vi "SerialCom_main.vi"(0 "VISA resource name":refnum<visa-resource-name>, 5 "write buffer":string, 11 "error in (no error)":errorcluster) -> (15 "error out":errorcluster)   [LabVIEW 2018]
uses:
  <vilib>/Instr/_visa.llb/VISA Flush IO Buffer Mask.ctl
  <vilib>/Instr/_visa.llb/VISA Configure Serial Port (Instr).vi
panel:
  out "binary[7]":string
  out "number[7]":u32
  out "byte[7]":string
  out "number[4]":u32
  out "number[5]":u32
  out "number[6]":u32
  out "binary[6]":string
  out "byte[6]":string
  out "binary[5]":string
  out "byte[5]":string
  out "byte[4]":string
  out "binary[4]":string
  in  "resetValues":bool
  out "binary[3]":string
  out "number[3]":u32
  out "byte[3]":string
  out "number[0]":u32
  out "number[1]":u32
  out "number[2]":u32
  out "binary[2]":string
  out "byte[2]":string
  out "binary[1]":string
  out "byte[1]":string
  out "byte[0]":string
  out "binary[0]":string
  out "byte Array":string[](array[string])
  out "valid byte":string
  out "bytes at port":u32
  out "byte count":u32
  out "read buffer":string
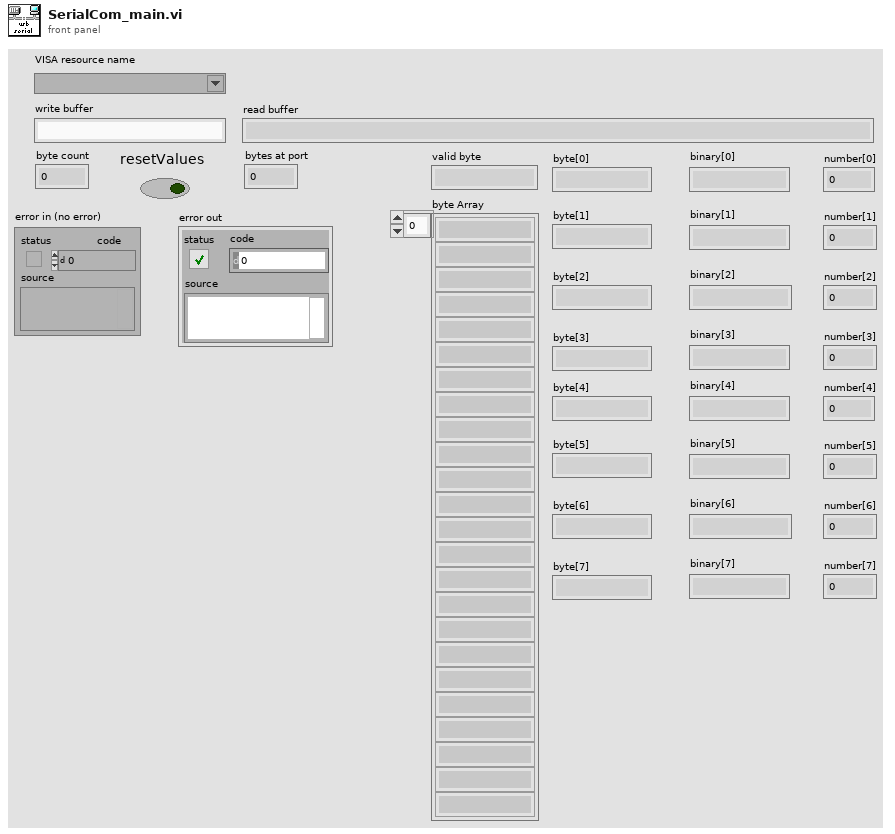
[diagram p1: front panel]
types:
  T1 = typedef "VISA Flush IO Buffer Mask.ctl" = u16
  T2 = cluster{"[0]":string, "[1]":string, "[2]":string, "[3]":string, "[4]":string, "[5]":string, "[6]":string, "[7]":string, "[8]":string}
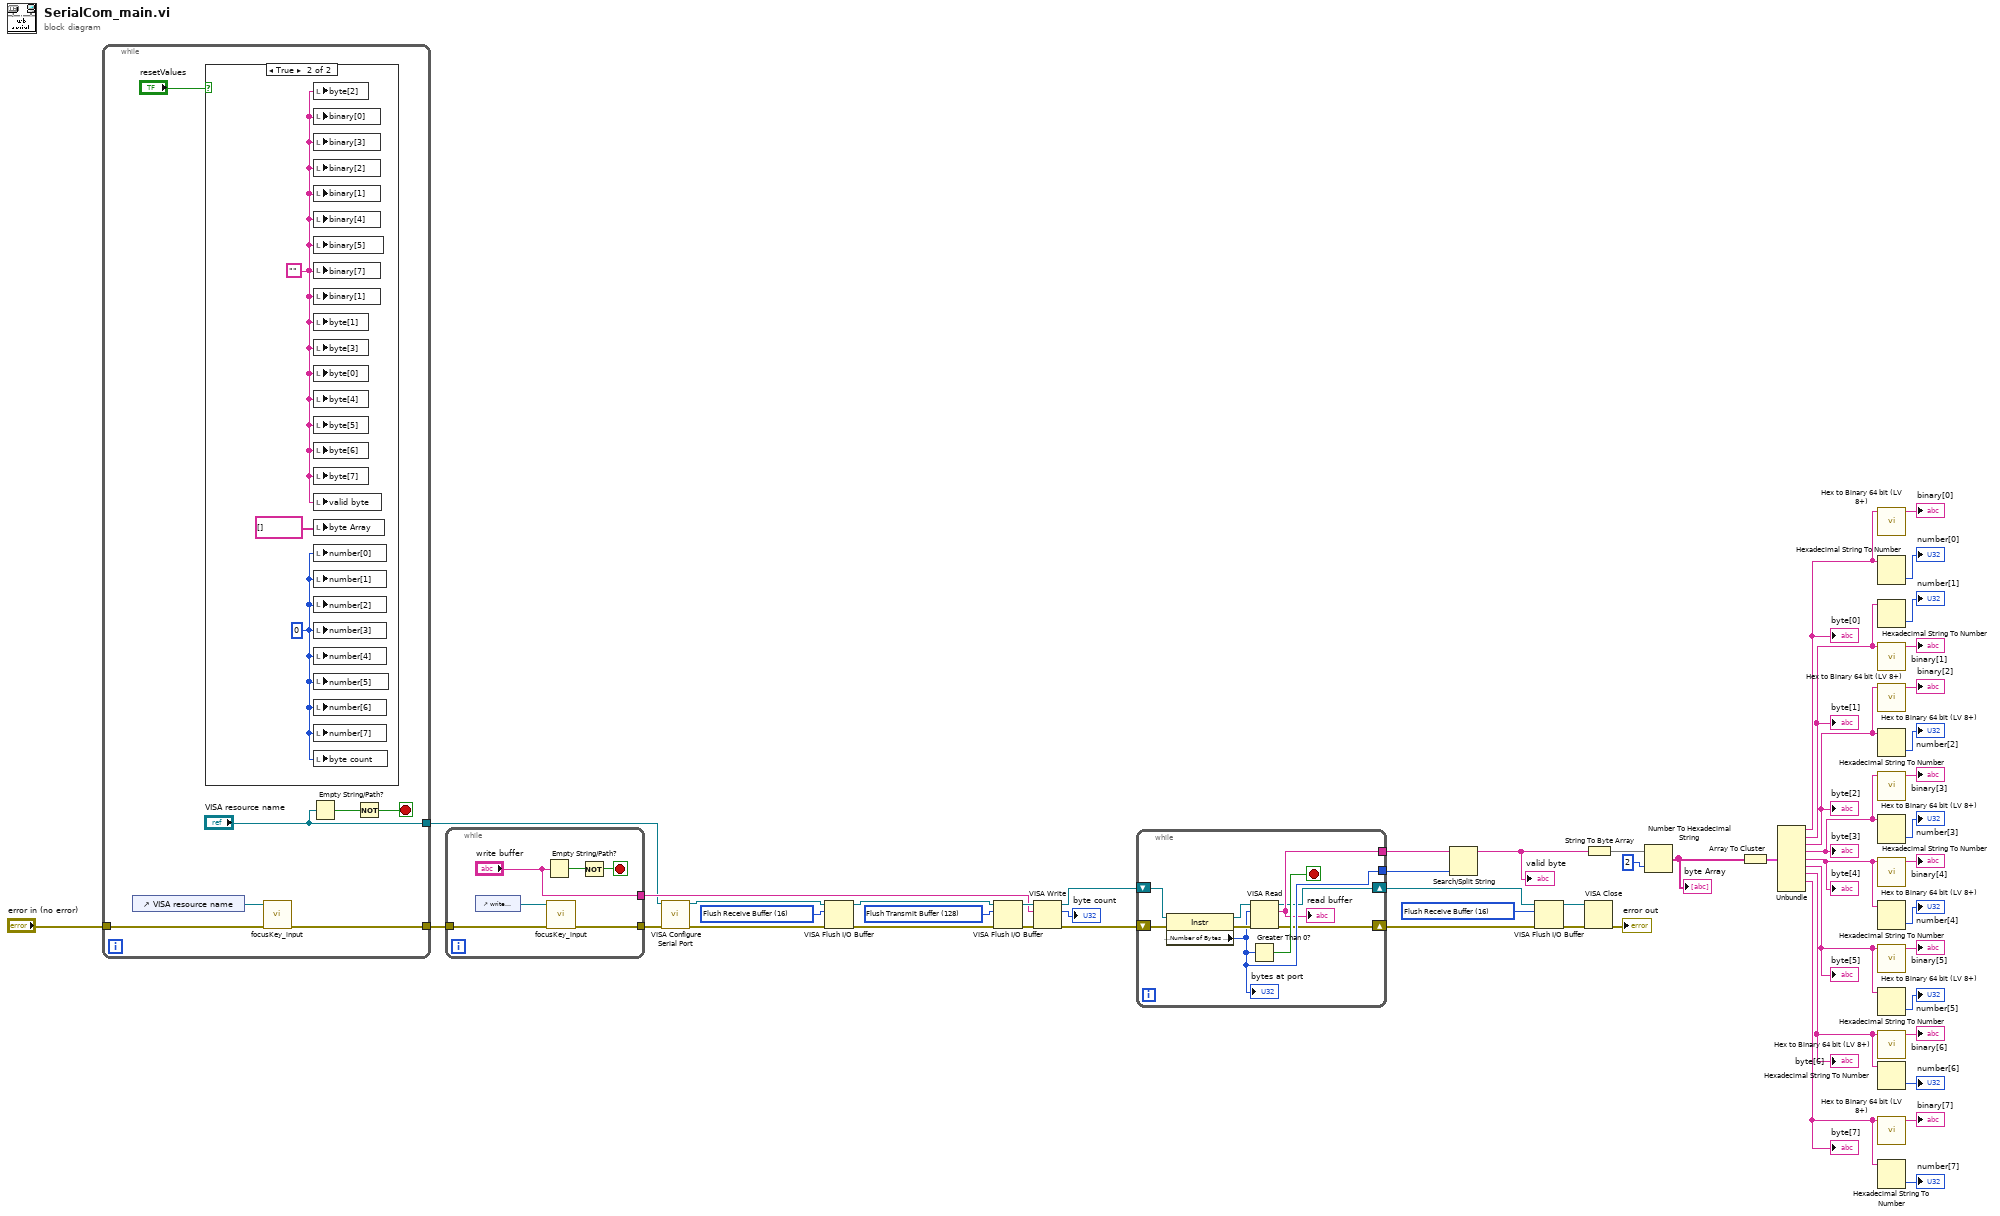
[diagram p0: block diagram]
diagram:
  w36 = T1 128 items=["Flush Receive Buffer"=16, "Write Transmit Buffer to Device"=32, "Flush Receive Buffer (No I/O)"=64, "Flush Transmit Buffer"=128] ("Mask")
  w40 = T1 16 items=["Flush Receive Buffer"=16, "Write Transmit Buffer to Device"=32, "Flush Receive Buffer (No I/O)"=64, "Flush Transmit Buffer"=128] ("Mask")
  w43 = T1 16 items=["Flush Receive Buffer"=16, "Write Transmit Buffer to Device"=32, "Flush Receive Buffer (No I/O)"=64, "Flush Transmit Buffer"=128] ("Mask")
  n1 = while {
    tunnel: ["VISA resource name"] -> w29
    tunnel: [w60] -> w28
    tunnel: "error in (no error)" -> [w59]
    stop <- w55 stop-if-true
    n2 = control-ref of="VISA resource name"() -> (w58:refnum<vi>)
    n3 = case shown="True" "resetValues" {
      frame False {
      }
      frame True {
        w62 = u32 0
        w61 = ""
        n4 = local write "byte[2]"(w61) -> ()
        n5 = local write "binary[0]"(w61) -> ()
        n6 = local write "binary[3]"(w61) -> ()
        n7 = local write "binary[2]"(w61) -> ()
        n8 = local write "binary[1]"(w61) -> ()
        n9 = local write "binary[4]"(w61) -> ()
        n10 = local write "binary[5]"(w61) -> ()
        n11 = local write "binary[7]"(w61) -> ()
        n12 = local write "binary[1]"(w61) -> ()
        n13 = local write "byte[1]"(w61) -> ()
        n14 = local write "byte[3]"(w61) -> ()
        n15 = local write "byte[0]"(w61) -> ()
        n16 = local write "byte[4]"(w61) -> ()
        n17 = local write "byte[5]"(w61) -> ()
        n18 = local write "byte[6]"(w61) -> ()
        n19 = local write "byte[7]"(w61) -> ()
        n20 = local write "valid byte"(w61) -> ()
        n21 = local write "byte Array"(string[] []) -> ()
        n22 = local write "number[0]"(w62) -> ()
        n23 = local write "number[1]"(w62) -> ()
        n24 = local write "number[2]"(w62) -> ()
        n25 = local write "number[3]"(w62) -> ()
        n26 = local write "number[4]"(w62) -> ()
        n27 = local write "number[5]"(w62) -> ()
        n28 = local write "number[6]"(w62) -> ()
        n29 = local write "number[7]"(w62) -> ()
        n30 = local write "byte count"(w62) -> ()
      }
    }
    n31 = call "focusKey_input.vi"("error in (no error)"=w59, "reference"=w58) -> ("error out"=w60:errorcluster)  [unwired: 9 in]
    n32 = Empty String/Path?(string/path="VISA resource name") -> (empty?=w56:bool)
    n33 = Not(x=w56) -> (.not. x?=w55:bool)
  }
  n34 = while {
    tunnel: ["write buffer"] -> w30
    tunnel: w28 -> [w69]
    tunnel: [w68] -> w27
    stop <- w64 stop-if-true
    n35 = control-ref of="write buffer"() -> (w67:refnum<vi>)
    n36 = Empty String/Path?(string/path="write buffer") -> (empty?=w65:bool)
    n37 = call "focusKey_input.vi"("error in (no error)"=w69, "reference"=w67) -> ("error out"=w68:errorcluster)  [unwired: 9 in]
    n38 = Not(x=w65) -> (.not. x?=w64:bool)
  }
  n39 = call-poly "VISA Configure Serial Port"("VISA resource name"=w29, "error in (no error)"=w27) -> ("VISA resource name out"=w42:refnum<visa-resource-name>, "error out"=w41:errorcluster)  [unwired: 12 in]
  n40 = VISA Flush I/O Buffer(VISA resource name=w42, mask (16)=w40, error in (no error)=w41) -> (VISA resource name out=w37:refnum<visa-resource-name>, error out=w38:errorcluster)
  n41 = VISA Flush I/O Buffer(VISA resource name=w37, mask (16)=w36, error in (no error)=w38) -> (VISA resource name out=w35:refnum<visa-resource-name>, error out=w34:errorcluster)
  n42 = VISA Write(VISA resource name=w35, write buffer=w30, error in (no error)=w34) -> (VISA resource name out=w53:refnum<visa-resource-name>, return count=→"byte count":u32, error out=w52:errorcluster)
  n43 = while {
    tunnel: [w72] -> w50
    tunnel: [w73] -> w47
    shift-right: [w70] -> w39
    shift-left: w53 -> [w78]
    shift-right: [w71] -> w44
    shift-left: w52 -> [w77]
    stop <- w74 stop-if-true
    n44 = property class="Instr"(reference=w78, error in=w77) -> (reference out=w75:refnum<visa-resource-name>, error out=w76:errorcluster, "Serial Settings:Number of Bytes at Serial Port"=w73:u32)
    "bytes at port" <- w73
    n45 = Greater Than 0?(x=w73) -> (x > 0?=w74:bool)
    n46 = VISA Read(VISA resource name=w75, byte count=w73, error in (no error)=w76) -> (VISA resource name out=w70:refnum<visa-resource-name>, read buffer=w72:string, error out=w71:errorcluster)  [unwired: 1 out]
    "read buffer" <- w72
  }
  n47 = Search/Split String(string=w50, offset (0)=w47) -> (substring before match=w45:string)  [unwired: 1 in, 2 out]
  "valid byte" <- w45
  n48 = VISA Flush I/O Buffer(VISA resource name=w39, mask (16)=w43, error in (no error)=w44) -> (VISA resource name out=w33:refnum<visa-resource-name>, error out=w32:errorcluster)
  n49 = String To Byte Array(string=w45) -> (unsigned byte array=w49:u8[])
  n50 = VISA Close(VISA resource name=w33, error in (no error)=w32) -> (error out=→"error out":errorcluster)
  n51 = Number To Hexadecimal String(1:i16 2 ("width (-)"), 2:w49) -> (0:w48:string[])
  "byte Array" <- w48
  n52 = Array To Cluster(array=w48) -> (cluster=w15:T2)
  n53 = Unbundle(w15) -> ("[0]"=w16:string, "[1]"=w17:string, "[2]"=w23:string, "[3]"=w13:string, "[4]"=w8:string, "[5]"=w7:string, "[6]"=w6:string, "[7]"=w5:string)  [unwired: 1 out]
  "byte[0]" <- w16
  "byte[1]" <- w17
  "byte[2]" <- w23
  "byte[3]" <- w13
  "byte[4]" <- w8
  "byte[5]" <- w7
  "byte[6]" <- w6
  "byte[7]" <- w5
  n54 = call "Hex to Binary 64 bit (LV 8+).vi"("Hexadecimal String"=w16) -> ("Binary String"=→"binary[0]":string)  [unwired: 6 in, 2 out]
  n55 = Hexadecimal String To Number(string=w16) -> (number=→"number[0]":u32)  [unwired: 2 in, 1 out]
  n56 = Hexadecimal String To Number(string=w17) -> (number=→"number[1]":u32)  [unwired: 2 in, 1 out]
  n57 = call "Hex to Binary 64 bit (LV 8+).vi"("Hexadecimal String"=w17) -> ("Binary String"=→"binary[1]":string)  [unwired: 6 in, 2 out]
  n58 = call "Hex to Binary 64 bit (LV 8+).vi"("Hexadecimal String"=w23) -> ("Binary String"=→"binary[2]":string)  [unwired: 6 in, 2 out]
  n59 = Hexadecimal String To Number(string=w23) -> (number=→"number[2]":u32)  [unwired: 2 in, 1 out]
  n60 = call "Hex to Binary 64 bit (LV 8+).vi"("Hexadecimal String"=w13) -> ("Binary String"=→"binary[3]":string)  [unwired: 6 in, 2 out]
  n61 = Hexadecimal String To Number(string=w13) -> (number=→"number[3]":u32)  [unwired: 2 in, 1 out]
  n62 = call "Hex to Binary 64 bit (LV 8+).vi"("Hexadecimal String"=w8) -> ("Binary String"=→"binary[4]":string)  [unwired: 6 in, 2 out]
  n63 = Hexadecimal String To Number(string=w8) -> (number=→"number[4]":u32)  [unwired: 2 in, 1 out]
  n64 = call "Hex to Binary 64 bit (LV 8+).vi"("Hexadecimal String"=w7) -> ("Binary String"=→"binary[5]":string)  [unwired: 6 in, 2 out]
  n65 = Hexadecimal String To Number(string=w7) -> (number=→"number[5]":u32)  [unwired: 2 in, 1 out]
  n66 = call "Hex to Binary 64 bit (LV 8+).vi"("Hexadecimal String"=w6) -> ("Binary String"=→"binary[6]":string)  [unwired: 6 in, 2 out]
  n67 = Hexadecimal String To Number(string=w6) -> (number=→"number[6]":u32)  [unwired: 2 in, 1 out]
  n68 = call "Hex to Binary 64 bit (LV 8+).vi"("Hexadecimal String"=w5) -> ("Binary String"=→"binary[7]":string)  [unwired: 6 in, 2 out]
  n69 = Hexadecimal String To Number(string=w5) -> (number=→"number[7]":u32)  [unwired: 2 in, 1 out]
